vi "Line Chart Test.vi"() -> ()   [LabVIEW 2020]
uses:
  Line Chart/Line Chart.xctl
panel:
  out "Line Chart":T1(xcontrol)
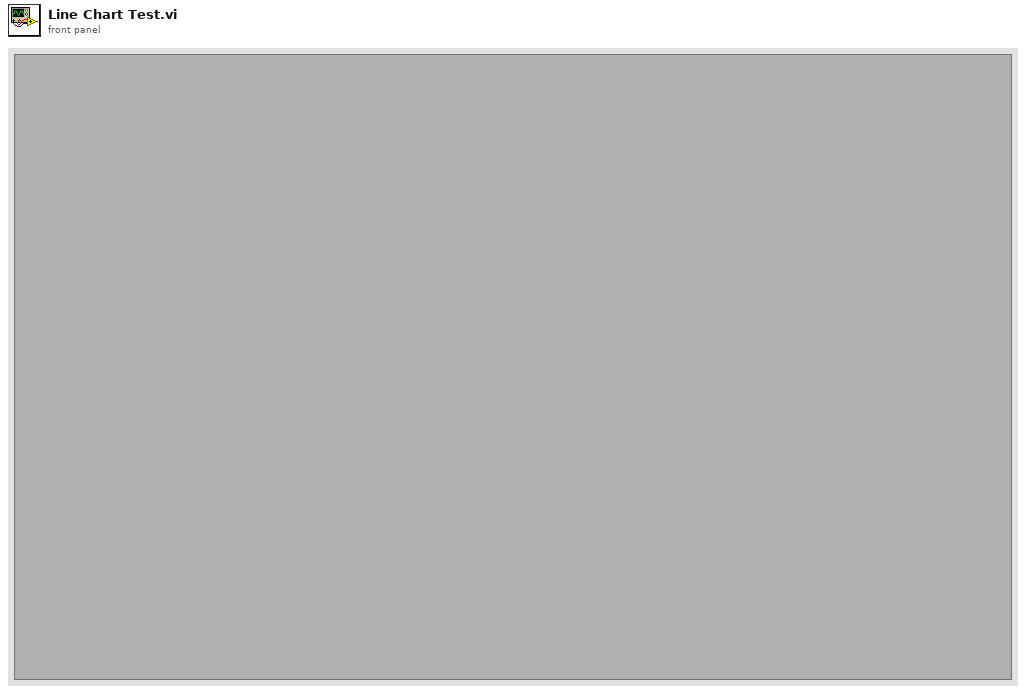
[diagram p1: front panel]
types:
  T1 = cluster{"X-Axis":string[], "Plots":cluster{"Data":dbl[], "Label":string, "Y-Axis":enum16{"Y-Axis 1", "Y-Axis 2"}, "Color":u32}[], "Plot Title":string}
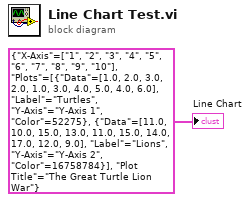
[diagram p0: block diagram]
diagram:
  "Line Chart" <- T1 {"X-Axis"=["1", "2", "3", "4", "5", "6", "7", "8", "9", "10"], "Plots"=[{"Data"=[1.0, 2.0, 3.0, 2.0, 1.0, 3.0, 4.0, 5.0, 4.0, 6.0], "Label"="Turtles", "Y-Axis"=enum."Y-Axis 1", "Color"=52275}, {"Data"=[11.0, 10.0, 15.0, 13.0, 11.0, 15.0, 14.0, 17.0, 12.0, 9.0], "Label"="Lions", "Y-Axis"=enum."Y-Axis 2", "Color"=16758784}], "Plot Title"="The Great Turtle Lion War"} ("Line Chart")
